vi "Deep Copy.vi"(8 "error in (no error)":errorcluster, 10 "Copy Actor In":refnum<class "System Actor.lvclass">, 11 "System Actor in":refnum<class "System Actor.lvclass">) -> (0 "error out":errorcluster, 2 "Coppied Actor Out":refnum<class "System Actor.lvclass">, 3 "System Actor out":refnum<class "System Actor.lvclass">)   [LabVIEW 2024, in "System Actor.lvclass"]
uses:
  System Actor.lvclass
  System Actor.lvclass/System Actor.ctl
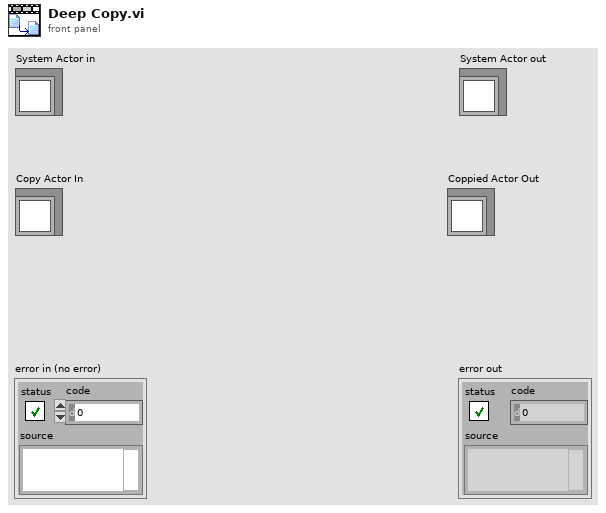
[diagram p1: front panel]
types:
  T1 = typedef "Rendezvous RefNum" = refnum<k1>
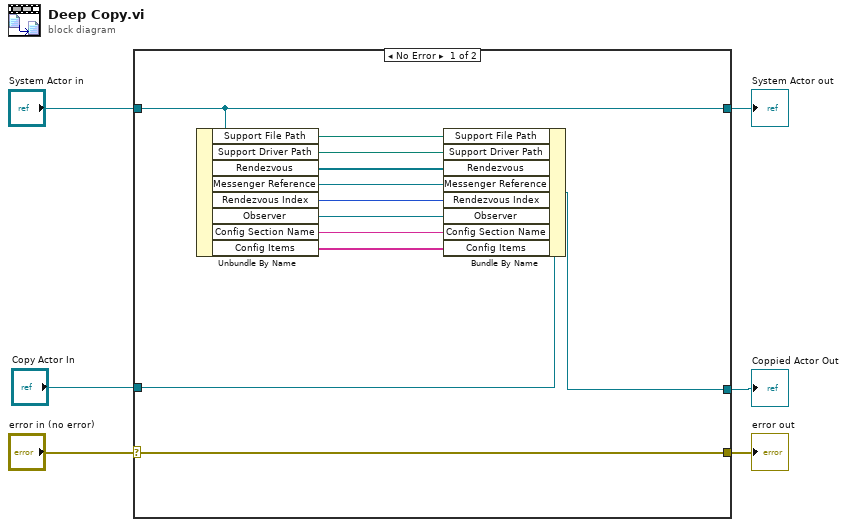
[diagram p0: block diagram]
diagram:
  n1 = case shown="No Error" "error in (no error)" {
    selector: "error in (no error)" -> [w18 w21]
    tunnel: [w18 w21] -> w5
    tunnel: [w17 w20] -> w3
    tunnel: "System Actor in" -> [w17 w20]
    tunnel: "Copy Actor In" -> [w16 w19]
    tunnel: [w7 w19] -> w1
    frame No Error {
      n2 = Unbundle By Name(w17) -> ("Support File Path"=w15:path, "Support Driver Path"=w14:path, "Rendezvous"=w13:T1[], "Messenger Reference"=w12:refnum<data-value>, "Rendezvous Index"=w11:i32, "Observer"=w10:refnum<class "Observer.lvclass">, "Config Section Name"=w9:string, "Config Items"=w8:string[])
      n3 = Bundle By Name(cluster=w16, "Support File Path"=w15, "Support Driver Path"=w14, "Rendezvous"=w13, "Messenger Reference"=w12, "Rendezvous Index"=w11, "Observer"=w10, "Config Section Name"=w9, "Config Items"=w8) -> (w7:refnum<class "System Actor.lvclass">)
    }
    frame Error {
    }
  }
  "error out" <- w5
  "System Actor out" <- w3
  "Coppied Actor Out" <- w1
